vi "串口助手 - 副本.vi"() -> ()   [LabVIEW 2013]
uses:
  <vilib>/Instr/_visa.llb/VISA Configure Serial Port (Instr).vi
  <vilib>/picture/picture.llb/Draw True-Color Pixmap.vi
panel:
  out "R分量":u8[][](array[numeric])
  out "G分量":u8[][](array[numeric])
  out "B分量":u8[][](array[numeric])
  in  "?":bool
  out "new picture 2":picture caption="新图片"
  in  "?":bool
  in  "接收16进制显示":bool
  in  "自动清空值：":string
  in  "自动清空接收区":bool
  in  "清空接收":bool
  out "接收总数":u32
  out "接收数目":u32
  out "接受错误状态":bool
  out "接收内容":string
  out "VISA资源名称输出":refnum<visa-resource-name>
  out "status":bool
  in  "波特率":u32(ring) caption="波特率选择" items=["4800"=4800, "9600"=9600, "115200"=115200, "128000"=128000]
  in  "串口号":refnum<visa-resource-name> caption="串口选择"
  in  "关闭串口":bool
  in  "打开串口":bool
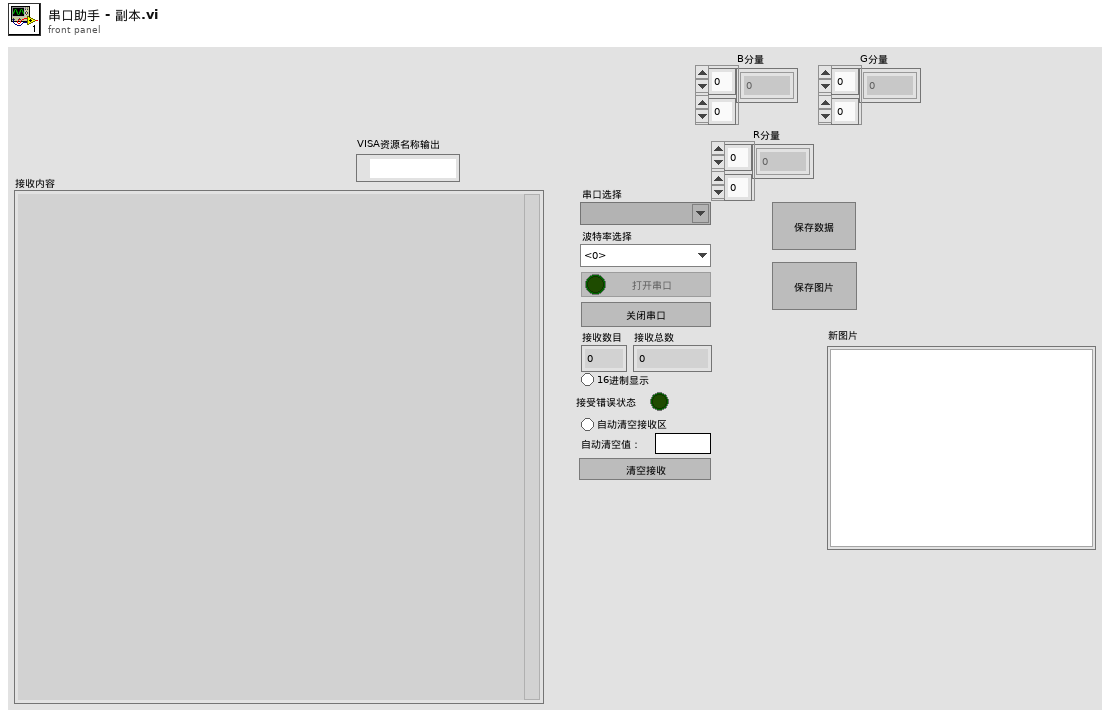
[diagram p1: front panel]
types:
  T1 = enum8{"Enabled", "Disabled", "Disabled and Grayed Out"}
  T2 = typedef "imagedata.ctl" = cluster{"image type":i32, "image depth":i32, "image":u8[], "mask":u8[], "colors":u32[], "Rectangle":cluster{"left":i16, "top":i16, "right":i16, "bottom":i16}}
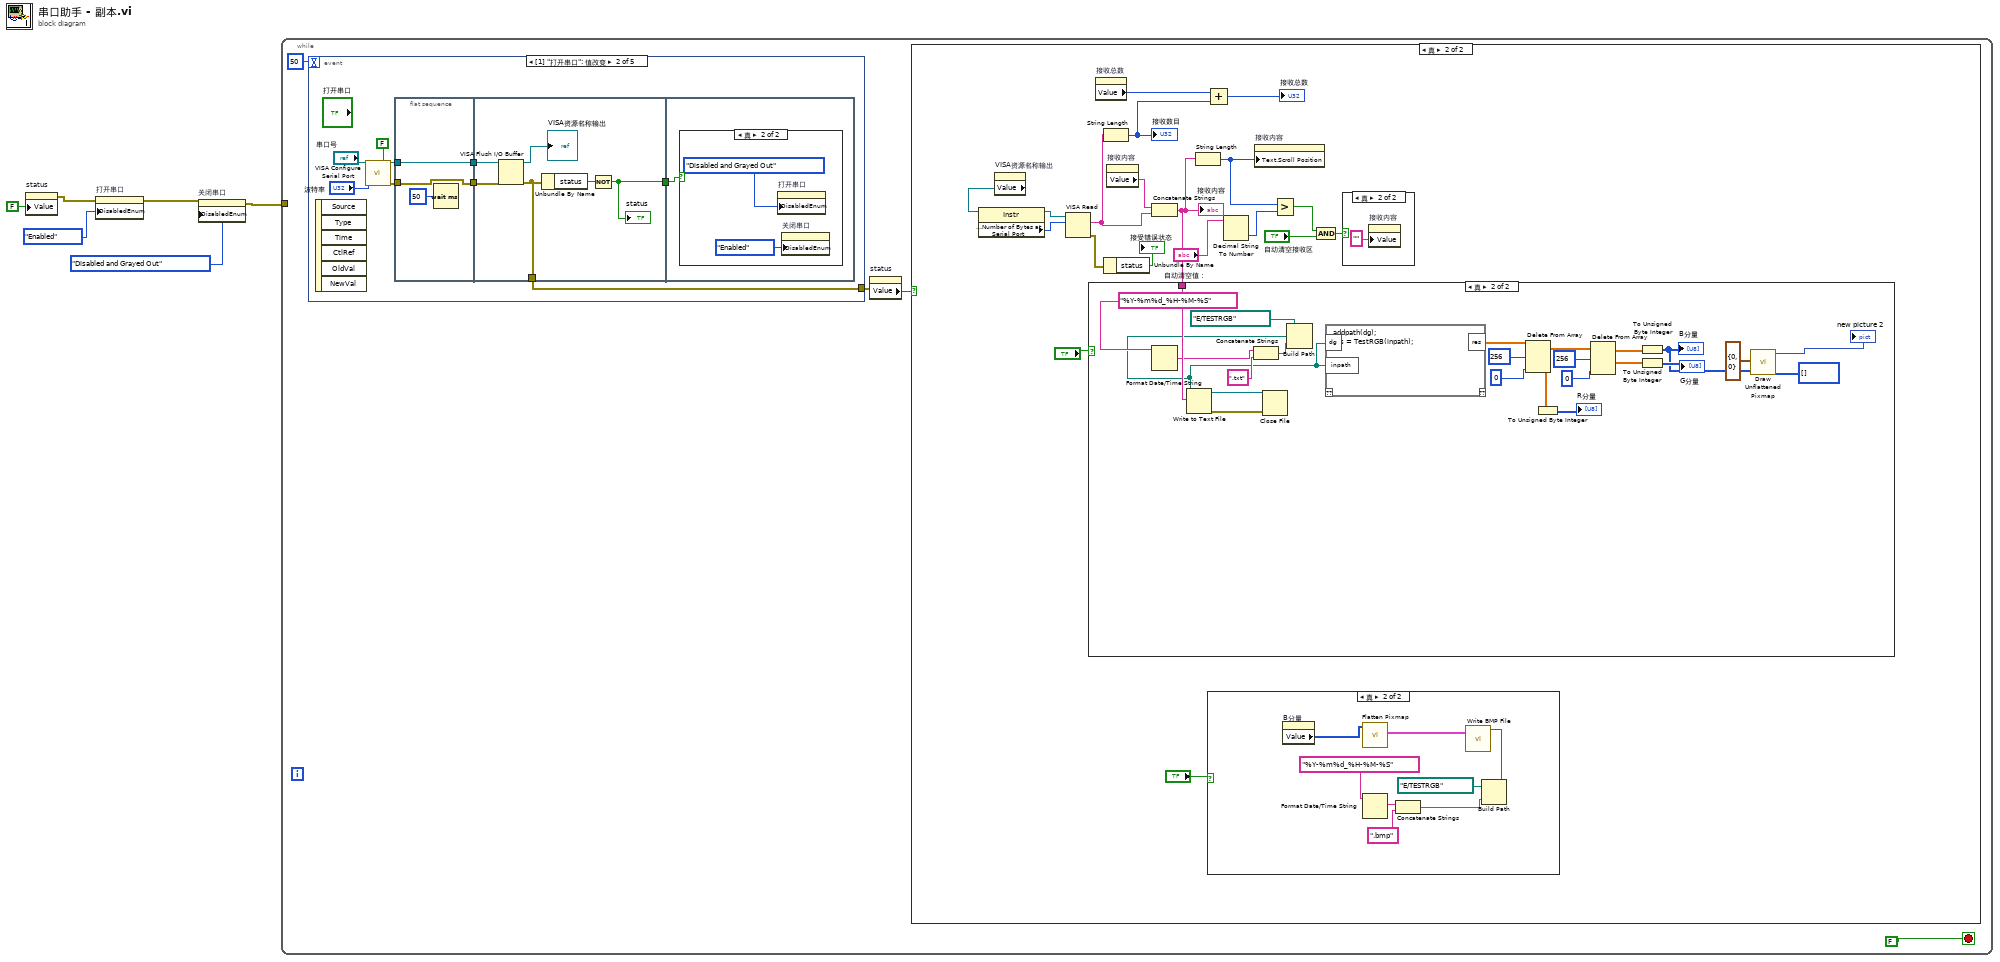
[diagram p0: block diagram]
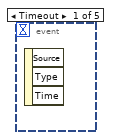
[diagram p6: hidden frame]
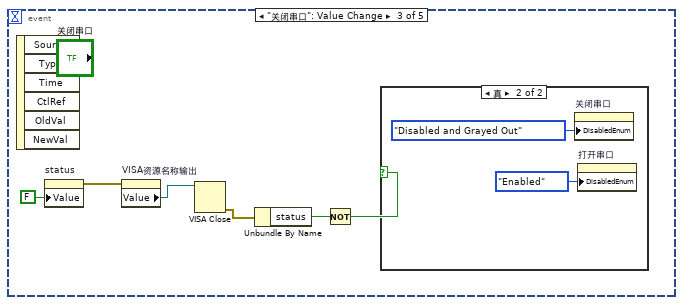
[diagram p8: hidden frame]
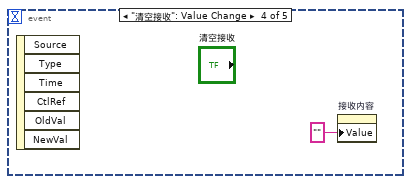
[diagram p10: hidden frame]
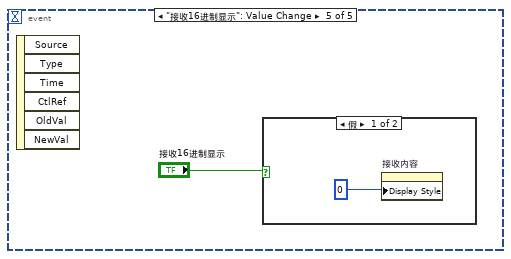
[diagram p11: hidden frame]
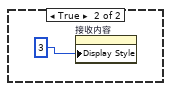
[diagram p12: hidden frame]
diagram:
  n1 = property on="status" class="Bool (严格)"("Value"=FALSE ("status")) -> (error out=w1:errorcluster)  [unwired: 2 in, 1 out]
  n2 = property on="打开串口" class="Bool"(error in=w1, "DisabledEnum"=T1."Enabled" ("禁用")) -> (error out=w4:errorcluster)  [unwired: 1 in, 1 out]
  n3 = property on="关闭串口" class="Bool"(error in=w4, "DisabledEnum"=T1."Disabled and Grayed Out" ("禁用")) -> (error out=w3:errorcluster)  [unwired: 1 in, 1 out]
  n4 = while {
    tunnel: w3 -> [_]
    stop <- FALSE stop-if-true
    n5 = event shown="[1] \"打开串口\": 值改变" {
      selector: _ -> [_ _ _ _ _]
      dyn-events: _ -> [_ _ _ _ _]
      timeout: 50 -> [_ _ _ _ _]
      tunnel: [_ w65 _ _ _] -> w8
      event Timeout {
        n6 = event-data() -> ()  [unwired: 1 in, 3 out]
      }
      event "打开串口": Value Change {
        n7 = event-data() -> ()  [unwired: 1 in, 6 out]
        n8 = call-poly "VISA Configure Serial Port"("VISA resource name"="串口号", "Enable Termination\nChar (T)"=FALSE ("Enable Termination\nChar (T)"), "baud rate (9600)"="波特率") -> ("VISA resource name out"=w70:refnum<visa-resource-name>, "error out"=w68:errorcluster)  [unwired: 11 in]
        n9 = flat-sequence {
          tunnel: w70 -> [w73]
          tunnel: [w73] -> w69
          tunnel: w68 -> [w72]
          tunnel: [w72] -> w67
          tunnel: w69 -> [w80]
          tunnel: w67 -> [w79]
          tunnel: [w77] -> w66
          tunnel: [w76] -> w65
          tunnel: w66 -> [w81]
          frame #0 {
            n10 = Wait (ms)(milliseconds to wait=u32 50 ("等待时间（毫秒）")) -> ()  [unwired: 1 out]
          }
          frame #1 {
            n11 = VISA Flush I/O Buffer(VISA resource name=w80, error in (no error)=w79) -> (VISA resource name out=→"VISA资源名称输出":refnum<visa-resource-name>, error out=w76:errorcluster)  [unwired: 1 in]
            n12 = Unbundle By Name(w76) -> ("status"=w78:bool)
            n13 = Not(x=w78) -> (.not. x?=w77:bool)
            "status" <- w77
          }
          frame #2 {
            n14 = case shown="真" w81 {
              frame False {
              }
              frame True {
                n15 = property on="打开串口" class="Bool"("DisabledEnum"=T1."Disabled and Grayed Out" ("禁用")) -> ()  [unwired: 2 in, 2 out]
                n16 = property on="关闭串口" class="Bool"("DisabledEnum"=T1."Enabled" ("禁用")) -> ()  [unwired: 2 in, 2 out]
              }
            }
          }
        }
      }
      event "关闭串口": Value Change {
        n17 = event-data() -> ()  [unwired: 1 in, 6 out]
        n18 = property on="status" class="Bool (严格)"("Value"=FALSE ("status")) -> (error out=w84:errorcluster)  [unwired: 2 in, 1 out]
        n19 = property on="VISA资源名称输出" class="VISAName"(error in=w84) -> ("Value"=w89:refnum<visa-resource-name>)  [unwired: 1 in, 2 out]
        n20 = VISA Close(VISA resource name=w89) -> (error out=w88:errorcluster)  [unwired: 1 in]
        n21 = Unbundle By Name(w88) -> ("status"=w87:bool)
        n22 = Not(x=w87) -> (.not. x?=w86:bool)
        n23 = case shown="真" w86 {
          frame False {
          }
          frame True {
            n24 = property on="关闭串口" class="Bool"("DisabledEnum"=T1."Disabled and Grayed Out" ("禁用")) -> ()  [unwired: 2 in, 2 out]
            n25 = property on="打开串口" class="Bool"("DisabledEnum"=T1."Enabled" ("禁用")) -> ()  [unwired: 2 in, 2 out]
          }
        }
      }
      event "清空接收": Value Change {
        n26 = event-data() -> ()  [unwired: 1 in, 6 out]
        n27 = property on="接收内容" class="Str"("Value"="" ("接收内容")) -> ()  [unwired: 2 in, 2 out]
      }
      event "接收16进制显示": Value Change {
        n28 = event-data() -> ()  [unwired: 1 in, 6 out]
        n29 = case shown="假" "接收16进制显示" {
          frame False {
            n30 = property on="接收内容" class="Str"("Display Style"=u32 0 ("显示样式")) -> ()  [unwired: 2 in, 2 out]
          }
          frame True {
            n31 = property on="接收内容" class="Str"("Display Style"=u32 3 ("显示样式")) -> ()  [unwired: 2 in, 2 out]
          }
        }
      }
    }
    n32 = property on="status" class="Bool (严格)"(error in=w8) -> ("Value"=w7:bool)  [unwired: 1 in, 2 out]
    n33 = case shown="真" w7 {
      frame False {
      }
      frame True {
        n34 = property on="VISA资源名称输出" class="VISAName"() -> ("Value"=w28:refnum<visa-resource-name>)  [unwired: 2 in, 2 out]
        n35 = property class="Instr"(reference=w28) -> (reference out=w29:refnum<visa-resource-name>, "Serial Settings:Number of Bytes at Serial Port"=w23:u32)  [unwired: 1 in, 1 out]
        n36 = VISA Read(VISA resource name=w29, byte count=w23) -> (read buffer=w14:string, error out=w26:errorcluster)  [unwired: 1 in, 2 out]
        n37 = property on="接收总数" class="DigNum (严格)"() -> ("Value"=w24:u32)  [unwired: 2 in, 2 out]
        n38 = String Length(string=w14) -> (length=w22:i32)
        "接收数目" <- w22
        n39 = Unbundle By Name(w26) -> ("status"=→"接受错误状态":bool)
        n40 = property on="接收内容" class="Str"() -> ("Value"=w16:string)  [unwired: 2 in, 2 out]
        n41 = Concatenate Strings(w16, w14) -> (w13:string)
        "接收内容" <- w13
        n42 = case shown="真" "?" {
          tunnel: w13 -> [_ w59]
          frame False {
          }
          frame True {
            n43 = Format Date/Time String(time format string (%c)="%Y-%m%d_%H-%M-%S" ("时间格式字符串(%c)")) -> (date/time string=w43:string)  [unwired: 2 in]
            n44 = Concatenate Strings(w43, ".txt" ("字符串")) -> (w42:string)
            n45 = Build Path(base path=path "E:/TESTRGB", name or relative path=w42) -> (appended path=w41:path)
            n46 = Write to Text File(file (use dialog)=w41, text=w59) -> (refnum out=w61:refnum<file>, error out=w60:errorcluster)  [unwired: 2 in, 1 out]
            n47 = Close File(refnum=w61, error in=w60) -> ()  [unwired: 2 out]
            n48 = script code="addpath(dg);\nres = TestRGB(inpath);"("inpath"=w41, "dg"=w41) -> ("res"=w48:dbl[][])  [unwired: 1 in, 1 out]
            n49 = Delete From Array(array=w48, length=256 ("长度"), index (col)=0 ("禁用的索引 (列)")) -> (deleted portion=w51:dbl[][], array with subset deleted=w54:dbl[][])  [unwired: 1 in]
            n50 = To Unsigned Byte Integer(number=w51) -> (unsigned 8bit integer=→"R分量":u8[][])
            n51 = Delete From Array(array=w54, length=256 ("长度"), index (col)=0 ("禁用的索引 (列)")) -> (deleted portion=w50:dbl[][], array with subset deleted=w49:dbl[][])  [unwired: 1 in]
            n52 = To Unsigned Byte Integer(number=w49) -> (unsigned 8bit integer=w38:u8[][])
            "B分量" <- w38
            n53 = To Unsigned Byte Integer(number=w50) -> (unsigned 8bit integer=→"G分量":u8[][])
            n54 = call-poly <vilib>:"Draw Unflattened Pixmap.vi"("top left point(0, 0)"=cluster{"x":i16, "y":i16} {"x"=0, "y"=0}, "data (RGB format)"=w38, "mask"=u8[] []) -> ("new picture"=→"new picture 2":picture)  [unwired: 6 in]
          }
        }
        n55 = String Length(string=w13) -> (length=w15:i32)
        n56 = Add(x=w24, y=w22) -> (x+y=→"接收总数":u32)
        n57 = case shown="真" "?" {
          frame False {
          }
          frame True {
            n58 = property on="B分量" class="Arr (严格)"() -> ("Value"=w30:u8[][])  [unwired: 2 in, 2 out]
            n59 = call <vilib>:"Flatten Pixmap.vi"("24-bit pixmap"=w30) -> ("image data"=w37:T2)  [unwired: 10 in]
            n60 = Format Date/Time String(time format string (%c)="%Y-%m%d_%H-%M-%S" ("时间格式字符串(%c)")) -> (date/time string=w32:string)  [unwired: 2 in]
            n61 = Concatenate Strings(w32, ".bmp" ("字符串")) -> (w35:string)
            n62 = Build Path(base path=path "E:/TESTRGB" ("基路径"), name or relative path=w35) -> (appended path=w33:path)
            n63 = call <vilib>:"Write BMP File.vi"("image data"=w37, "path to BMP file"=w33) -> ()  [unwired: 8 in, 2 out]
          }
        }
        n64 = Decimal String To Number(string="自动清空值：") -> (number=w17:i32)  [unwired: 2 in, 1 out]
        n65 = property on="接收内容" class="Str"("Text.Scroll Position"=w15) -> ()  [unwired: 2 in, 2 out]
        n66 = Greater?(x=w15, y=w17) -> (0:w21:bool)
        n67 = And(x=w21, y="自动清空接收区") -> (x .and. y?=w19:bool)
        n68 = case shown="真" w19 {
          frame False {
          }
          frame True {
            n69 = property on="接收内容" class="Str"("Value"="" ("接收内容")) -> ()  [unwired: 2 in, 2 out]
          }
        }
      }
    }
  }
